vi "CostCalculation.vi"(8 "PrevisouCost":u64, 9 "Direction":T4, 10 "Position":T2, 11 "CostIn":T3(c390)) -> (0 "CostLowerOrTheSame":bool, 1 "Cost":T1, 2 "CostLower":bool, 3 "CostOut":T3(c390))   [LabVIEW 2023, in "2024_18.lvclass"]
uses:
  2024_18.lvclass
  <vilib>/Utility/miscctls.llb/LVMapReplaceAction.ctl
  Common/AOC_Direction.ctl
  Common/AOC_XY(I32).ctl
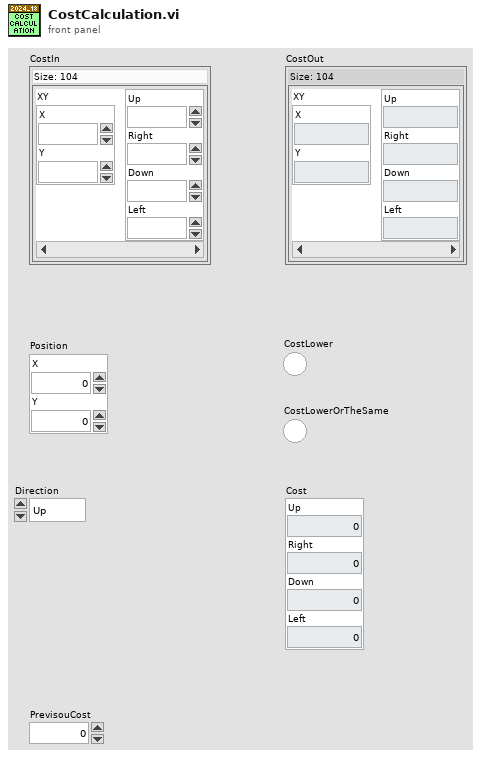
[diagram p1: front panel]
types:
  T1 = cluster{"Up":u64, "Right":u64, "Down":u64, "Left":u64}
  T2 = typedef "AOC_XY(I32).ctl" = cluster{"X":i32, "Y":i32}
  T3 = map{T2, cluster{"Up":u64, "Right":u64, "Down":u64, "Left":u64}}
  T4 = typedef "AOC_Direction.ctl" = enum16{"Up", "Right", "Down", "Left"}
  T5 = typedef "LVMapReplaceAction.ctl" = enum32{"Modify Entry only if found", "Add or Modify Entry", "Delete Entry"}
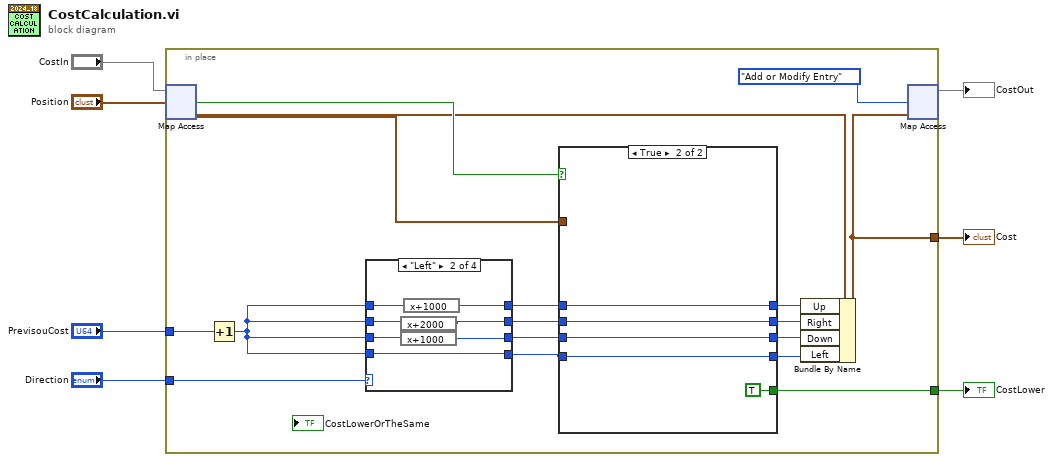
[diagram p0: block diagram]
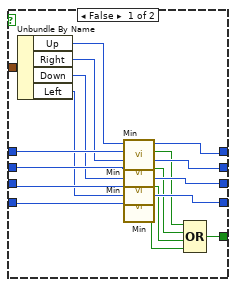
[diagram p2: hidden frame]
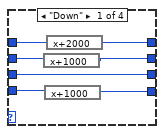
[diagram p3: hidden frame]
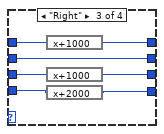
[diagram p4: hidden frame]
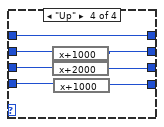
[diagram p5: hidden frame]
diagram:
  n1 = in-place {
    in-place-border: "Direction" -> [w23]
    in-place-border: "PrevisouCost" -> [w12]
    in-place-border: [w10] -> w3
    in-place-border: [w9] -> w2
    n2 = in-place-map #1("CostIn", "Position") -> (w13:T1, w22:bool)  [unwired: 1 in]
    n3 = Increment(x=w12) -> (x+1=w11:u64)
    n4 = case shown="\"Left\"" w23 {
      tunnel: w11 -> [w53 w60 w66 w68]
      tunnel: [w52 w59 w65 w68] -> w21
      tunnel: w11 -> [w51 w58 w67 w74]
      tunnel: [w50 w57 w67 w73] -> w20
      tunnel: w11 -> [w49 w55 w64 w70]
      tunnel: [w49 w54 w63 w69] -> w19
      tunnel: w11 -> [w48 w56 w62 w72]
      tunnel: [w47 w56 w61 w71] -> w18
      frame "Down" {
        n5 = expression code="x+1000"(w51) -> (w50:u64)
        n6 = expression code="x+1000"(w48) -> (w47:u64)
        n7 = expression code="x+2000"(w53) -> (w52:u64)
      }
      frame "Left" {
        n8 = expression code="x+2000"(w58) -> (w57:u64)
        n9 = expression code="x+1000"(w55) -> (w54:u64)
        n10 = expression code="x+1000"(w60) -> (w59:u64)
      }
      frame "Right" {
        n11 = expression code="x+1000"(w66) -> (w65:u64)
        n12 = expression code="x+1000"(w64) -> (w63:u64)
        n13 = expression code="x+2000"(w62) -> (w61:u64)
      }
      frame "Up" {
        n14 = expression code="x+1000"(w74) -> (w73:u64)
        n15 = expression code="x+2000"(w70) -> (w69:u64)
        n16 = expression code="x+1000"(w72) -> (w71:u64)
      }
    }
    n17 = case shown="True" w22 {
      tunnel: w21 -> [w41 w46]
      tunnel: w20 -> [w38 w45]
      tunnel: w19 -> [w35 w44]
      tunnel: w18 -> [w34 w43]
      tunnel: [w32 w46] -> w17
      tunnel: [w31 w45] -> w16
      tunnel: [w30 w44] -> w15
      tunnel: [w29 w43] -> w14
      tunnel: w13 -> [w40 _]
      tunnel: [w24 TRUE] -> w10
      frame False {
        n18 = Unbundle By Name(w40) -> ("Up"=w39:u64, "Right"=w37:u64, "Down"=w36:u64, "Left"=w33:u64)
        n19 = call "Min.vi"("Value 2"=w41, "Value 1"=w39) -> ("Value2 Smaller"=w28:bool, "Min value"=w32:u64)  [unwired: 8 in]
        n20 = call "Min.vi"("Value 2"=w38, "Value 1"=w37) -> ("Value2 Smaller"=w27:bool, "Min value"=w31:u64)  [unwired: 8 in]
        n21 = call "Min.vi"("Value 2"=w35, "Value 1"=w36) -> ("Value2 Smaller"=w26:bool, "Min value"=w30:u64)  [unwired: 8 in]
        n22 = call "Min.vi"("Value 2"=w34, "Value 1"=w33) -> ("Value2 Smaller"=w25:bool, "Min value"=w29:u64)  [unwired: 8 in]
        n23 = Compound Arithmetic op=OR(w28, w27, w26, w25) -> (w24:bool)
      }
      frame True {
      }
    }
    n24 = Bundle By Name(cluster=w13, "Up"=w17, "Right"=w16, "Down"=w15, "Left"=w14) -> (w9:T1)
    n25 = in-place-map #1(w9, LVMapReplaceAction."Add or Modify Entry" ("action")) -> (→"CostOut":T3)  [unwired: 2 out]
  }
  "Cost" <- w2
  "CostLower" <- w3
